vi "Supply_ComplianceCheck.vi"(8 "error in (no error)":errorcluster, 11 "KE237 in":refnum<class "KE237.lvclass">) -> (0 "error out":errorcluster, 1 "Status string":string, 2 "Compliance exceeded?":bool, 3 "KE237 out":refnum<class "KE237.lvclass">)   [LabVIEW 2018, in "KE237.lvclass"]
uses:
  KE237.lvclass
  <vilib>/regexp/Match Regular Expression.xnode
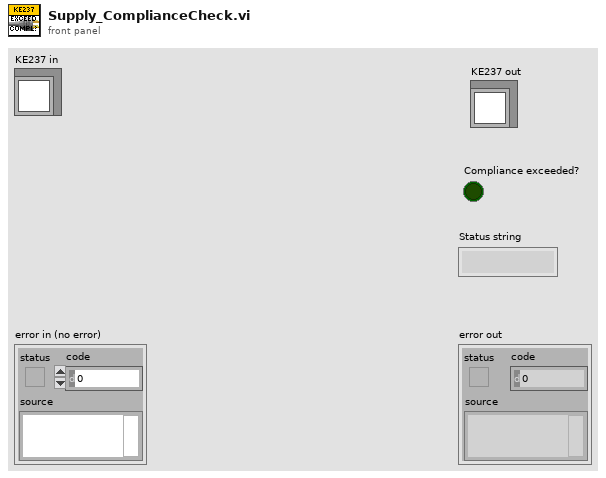
[diagram p1: front panel]
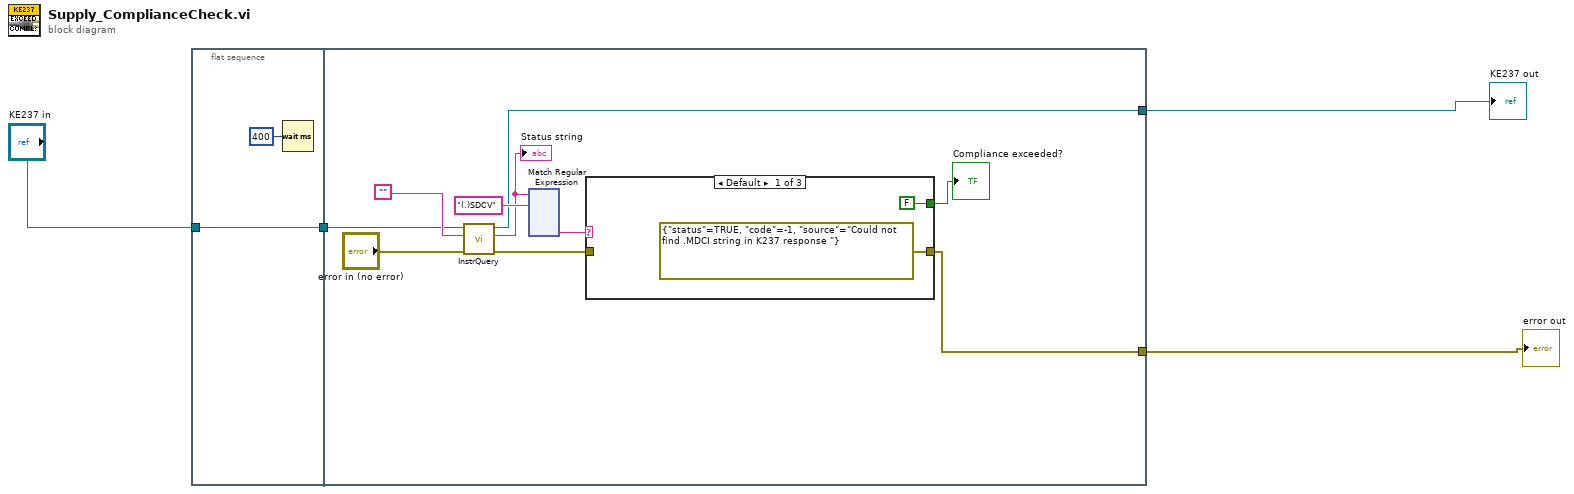
[diagram p0: block diagram]
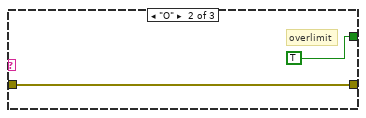
[diagram p2: hidden frame]
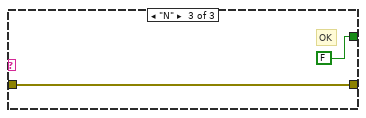
[diagram p3: hidden frame]
diagram:
  n1 = flat-sequence {
    tunnel: "KE237 in" -> [w6]
    tunnel: [w6] -> w1
    tunnel: w1 -> [w9]
    tunnel: [w8] -> w3
    tunnel: [w7] -> w2
    frame #0 {
      n2 = Wait (ms)(milliseconds to wait=u32 400) -> ()  [unwired: 1 out]
    }
    frame #1 {
      n3 = call-dynamic "InstrQuery.vi"("error in (no error)"="error in (no error)", "Command string"="", "InstControl in"=w9) -> ("error out"=w13:errorcluster, "Instrument response"=w14:string, "InstControl out"=w8:refnum<class "KE237.lvclass">)  [unwired: 6 in]
      "Status string" <- w14
      n4 = xnode "Match Regular Expression"("input string"=w14, "regular expression"="(.)SDCV") -> ("submatch 1"=w15:string)  [unwired: 4 in, 5 out]
      n5 = case shown="Default" w15 {
        tunnel: [FALSE ("Compliance exceeded?") TRUE ("Compliance exceeded?") FALSE ("Compliance exceeded?")] -> w11
        tunnel: [errorcluster {"status"=TRUE, "code"=-1, "source"="Could not find .MDCI string in K237 response "} ("error out") w19 w21] -> w7
        tunnel: w13 -> [_ w19 w21]
        frame Default {
        }
        frame "O" {
          # "overlimit"
        }
        frame "N" {
          # "OK"
        }
      }
      "Compliance exceeded?" <- w11
    }
  }
  "KE237 out" <- w3
  "error out" <- w2
